vi "icpcon_data_acquisition_loop_01_01.vi"(7 "sampling period (s)":dbl caption="采用周期 (s)", 8 "error in (no error)":errorcluster caption="错误输入（无错误）", 11 "Message Queues":T1 caption="消息队列") -> (0 "error out":errorcluster caption="错误输出")   [LabVIEW 2015]
uses:
  message_queue/all_rt_message_queues.ctl
  message_queue/message_cluster.ctl
  <vilib>/Platform/TimedLoop/XDataNode/timing_clust.ctl
  <vilib>/Platform/TimedLoop/XDataNode/nitl_modes.ctl
  <vilib>/Platform/TimedLoop/XDataNode/wakeup.ctl
  <vilib>/Instr/_visa.llb/VISA Configure Serial Port (Instr).vi
  <vilib>/Platform/TimedLoop/XDataNode/loadnilvce.vi
  globals/global_all_rt_loop_stop.vi
  <vilib>/Platform/TimedLoop/XDataNode/XDataNode.xnode
  <vilib>/Platform/TimedLoop/XDataNode/XDNodeRunTimeDep.lvlib
  message_queue/message_queue.lvlib
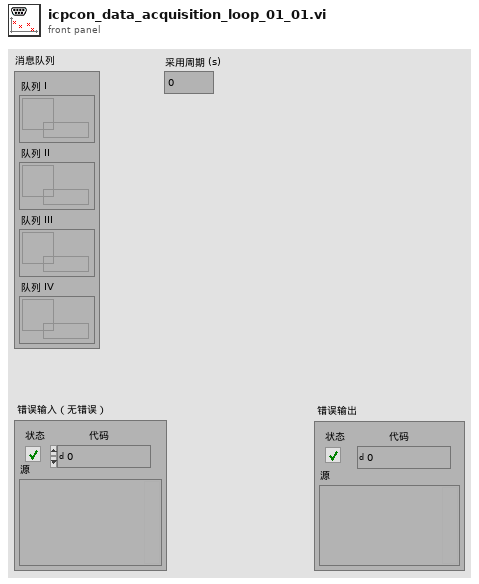
[diagram p1: front panel]
types:
  T1 = typedef "message_queue.lvlib/all_rt_message_queues.ctl" = cluster{"Queue I":refnum<queue>, "Queue II":refnum<queue>, "Queue III":refnum<queue>, "Queue IV":refnum<queue>}
  T2 = typedef "XDNodeRunTimeDep.lvlib/timing_clust.ctl" = cluster{"Expected End [f-1]":u64, "Actual End [f-1]":u64, "Finished Late? [f-1]":bool, "Expected End [i-1]":u64, "Actual End [i-1]":u64, "Finished Late? [i-1]":bool, "Expected Start [i]":u64, "Actual Start [i]":u64, "Expected Start [f]":u64, "Actual Start [f]":u64, "Source Name":string, "Structure Name":string, "Period":i64, "Deadline":i64, "Offset":i64, "Start":i64, "Priority":i32, "Timeout":i32, "Mode":T3, "Wakeup Reason":T4, "Error":errorcluster, "Source Type":string, "Secondary Source Type":string, "Global End Time":u64, "Global Start Time":u64, "Frame Duration":u64, "Iteration Duration":u64, "Assigned CPU":i32, "I/O Scan Engine Mode":u32}
  T3 = typedef "XDNodeRunTimeDep.lvlib/nitl_modes.ctl" = enum32{"No Change", "Process missed periods, maintain original phase", "Discard missed periods, maintain original phase", "Process missed periods, ignore original phase", "Discard missed periods, ignore original phase"}
  T4 = typedef "XDNodeRunTimeDep.lvlib/wakeup.ctl" = enum32{"Normal", "Aborted", "Asynchronous wakeup", "Timing source error", "Timed loop error", "Timeout"}
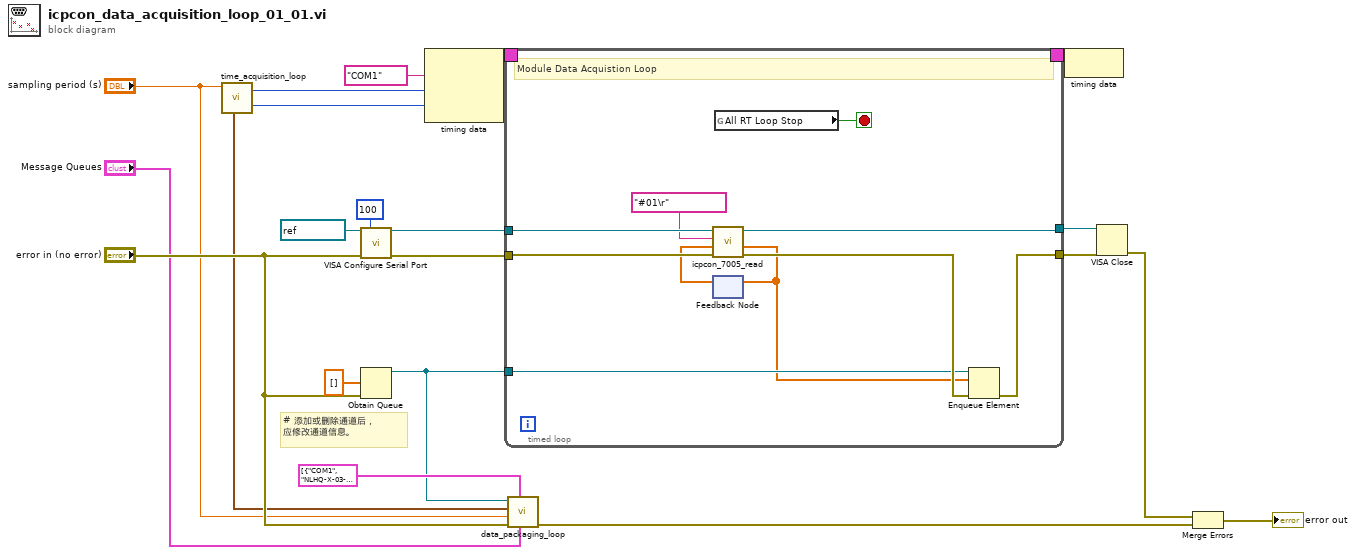
[diagram p0: block diagram]
diagram:
  # "# 添加或删除通道后，\n应修改通道信息。"
  n1 = call "time_acquisition_loop.vi"("Period (s)"="sampling period (s)") -> ("t0 (scan)"=w2:i64, "Period (scan)"=w3:i64, "timestamp output"=w1:timestamp)  [unwired: 4 in]
  n2 = call-poly "VISA Configure Serial Port"("VISA resource name"=refnum<visa-resource-name> "COM1", "timeout (10sec)"=u32 100, "error in (no error)"="error in (no error)") -> ("VISA resource name out"=w14:refnum<visa-resource-name>, "error out"=w5:errorcluster)  [unwired: 11 in]
  n3 = Obtain Queue(element data type=dbl[] [] ("数据类型"), error in (no error)="error in (no error)") -> (queue out=w7:refnum<queue>)  [unwired: 3 in, 2 out]
  n4 = node-c288("COM1" ("Structure Name"), w3, w2) -> (w20:T2)
  n5 = timed-loop {
    timing: w20 -> [_]
    timing-out: [_] -> w19
    tunnel: w7 -> [w23]
    tunnel: w5 -> [w29]
    tunnel: [w30] -> w16
    tunnel: [w26] -> w17
    tunnel: w14 -> [w28]
    stop <- w31 stop-if-true
    # "Module Data Acquistion Loop"
    n6 = feedback #1() -> (w27:dbl[])  [unwired: 1 in]
    n7 = call "icpcon_7005_read.vi"("error in (no error)"=w29, "Last Data Array"=w27, "write buffer"="#01\r", "VISA Ref Input"=w28) -> ("error out"=w25:errorcluster, "New Data Array"=w22:dbl[], "VISA Ref Output"=w26:refnum<visa-resource-name>)  [unwired: 5 in]
    n8 = feedback-in #1(w22) -> ()
    n9 = global read "global_all_rt_loop_stop.vi" "All RT Loop Stop"() -> (w31:bool)
    n10 = Enqueue Element(queue=w23, element=w22, error in (no error)=w25) -> (error out=w30:errorcluster)  [unwired: 1 in, 2 out]
  }
  n11 = call "data_packaging_loop.vi"("Message Queues"="Message Queues", "channel info array"=cluster{"Module":string, "Channel":string}[] [{"Module"="COM1", "Channel"="NLHQ-X-03-T01"}, {"Module"="COM1", "Channel"="NLHQ-X-03-T02"}, {"Module"="COM1", "Channel"="NLHQ-X-03-T03"}, {"Module"="COM1", "Channel"="NLHQ-X-03-T04"}, {"Module"="COM1", "Channel"="NLHQ-X-03-T05"}, {"Module"="COM1", "Channel"="NLHQ-X-03-T06"}, {"Module"="COM1", "Channel"="NLHQ-X-03-T07"}, {"Module"="COM1", "Channel"="NLHQ-X-03-T08"}], "error in (no error)"="error in (no error)", "sampling period (s)"="sampling period (s)", "timestamp"=w1, "data queue"=w7) -> ("error out"=w8:errorcluster)  [unwired: 5 in]
  n12 = node-c288(w19) -> ()
  n13 = VISA Close(VISA resource name=w17, error in (no error)=w16) -> (error out=w15:errorcluster)
  n14 = Merge Errors(w15, w8) -> (→"error out":errorcluster)
